vi "Error test.vi"() -> ()   [LabVIEW 2017, in "Error.lvlib"]
uses:
  Error.lvlib
panel:
  in  "Text":string
  in  "Kill":bool
  in  "error in (no error)":errorcluster
  in  "add":bool
  in  "stop":bool
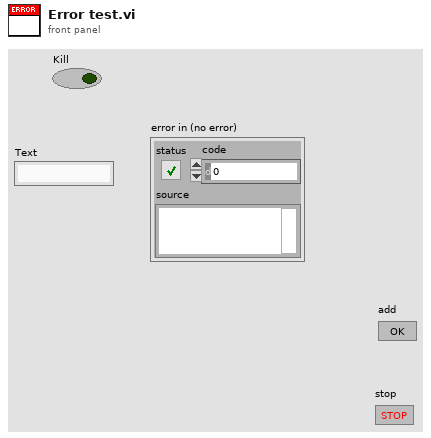
[diagram p1: front panel]
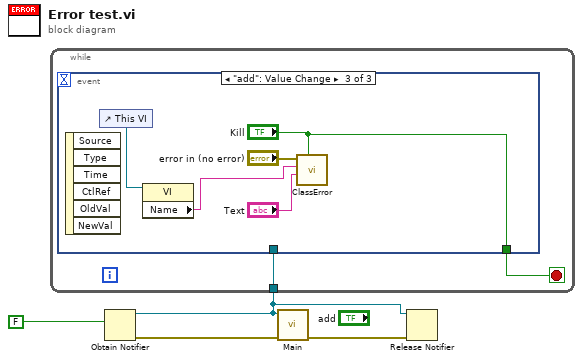
[diagram p0: block diagram]
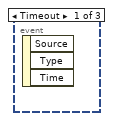
[diagram p2: hidden frame]
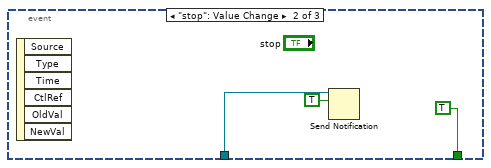
[diagram p3: hidden frame]
diagram:
  n1 = Obtain Notifier(notification data type=FALSE) -> (notifier out=w1:refnum<notifier>, error out=w3:errorcluster)  [unwired: 3 in, 1 out]
  n2 = while {
    tunnel: w1 -> [w6]
    stop <- w5 stop-if-true
    n3 = event shown="[2] \"add\": Value Change" {
      selector: _ -> [_ _ _]
      dyn-events: _ -> [_ _ _]
      timeout: _ -> [_ _ _]
      tunnel: w6 -> [_ w9 _]
      tunnel: [_ TRUE "Kill"] -> w5
      event Timeout {
        n4 = event-data() -> ()  [unwired: 1 in, 3 out]
      }
      event "stop": Value Change {
        n5 = event-data() -> ()  [unwired: 1 in, 6 out]
        n6 = Send Notification(notification=TRUE, notifier=w9) -> ()  [unwired: 1 in, 2 out]
      }
      event "add": Value Change {
        n7 = event-data() -> ()  [unwired: 1 in, 6 out]
        n8 = control-ref of="This VI"() -> (w11:refnum<vi>)
        n9 = property class="VI"(reference=w11) -> ("Name"=w10:string)  [unwired: 1 in, 2 out]
        n10 = call "ClassError.vi"("Kill"="Kill", "Text"="Text", "From"=w10, "error in"="error in (no error)") -> ()  [unwired: 7 in, 1 out]
      }
    }
  }
  n11 = call "Main.vi"("error in (no error)"=w3, "Stop notifier"=w1) -> ("error out"=w2:errorcluster)  [unwired: 9 in]
  n12 = Release Notifier(notifier=w1, error in (no error)=w2) -> ()  [unwired: 1 in, 3 out]
